vi "BT-Android_AE_sub.vi"(5 "mode":T1, 6 "timeout (10sec)":u32=10000, 7 "End Write on Termination Character?":bool, 8 "error in (no error)":errorcluster, 10 "send data":string, 11 "VISA resource name":refnum<visa-resource-name>="COM13") -> (0 "error IO":errorcluster, 2 "timeout?":bool=TRUE)   [LabVIEW 2016, in "BT-Android_interface.lvlib"]
uses:
  BT-Android_interface.lvlib
  mode.ctl
  <vilib>/Instr/_visa.llb/VISA Configure Serial Port (Instr).vi
panel:
  out "Bytes Remain":u32
  in  "Termination Character":u8=10 format="%.0x"
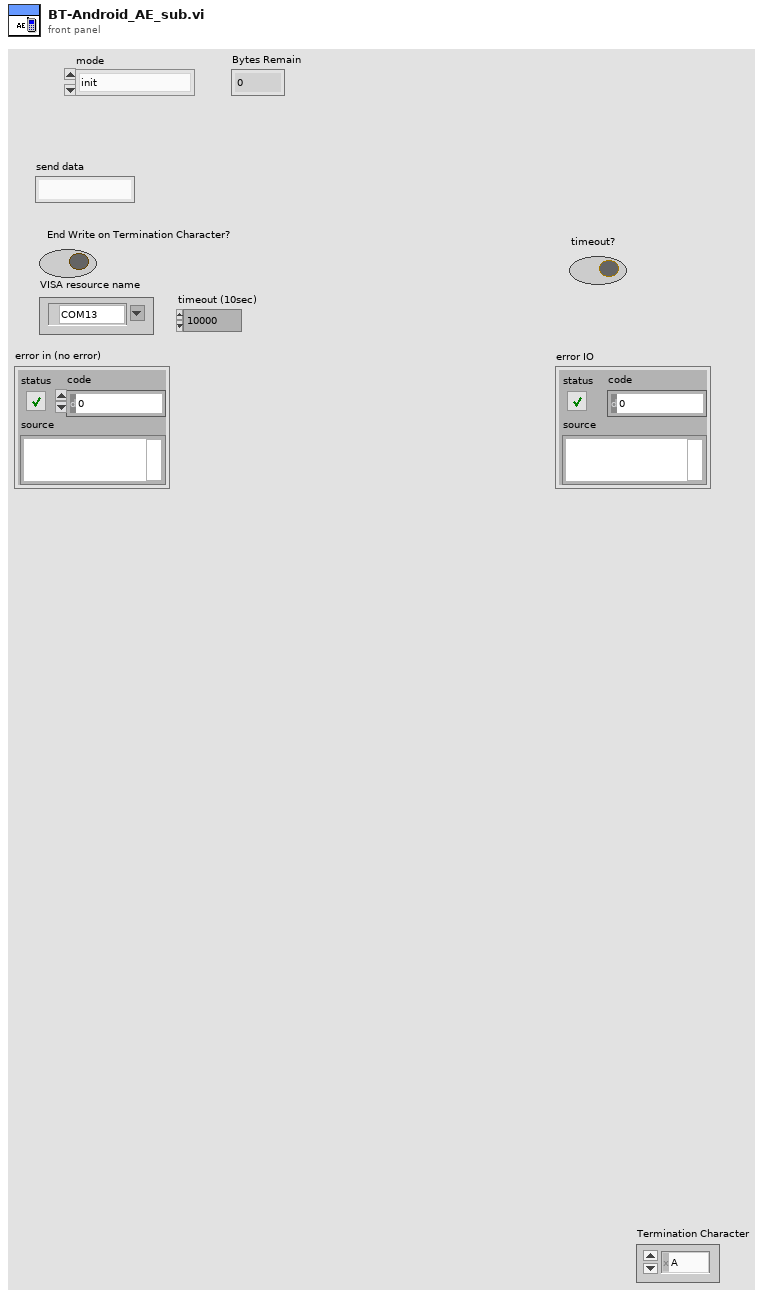
[diagram p1: front panel]
types:
  T1 = typedef "BT-Android_interface.lvlib/mode.ctl" = enum16{"init", "broadcast_data", "receive_data", "close"}
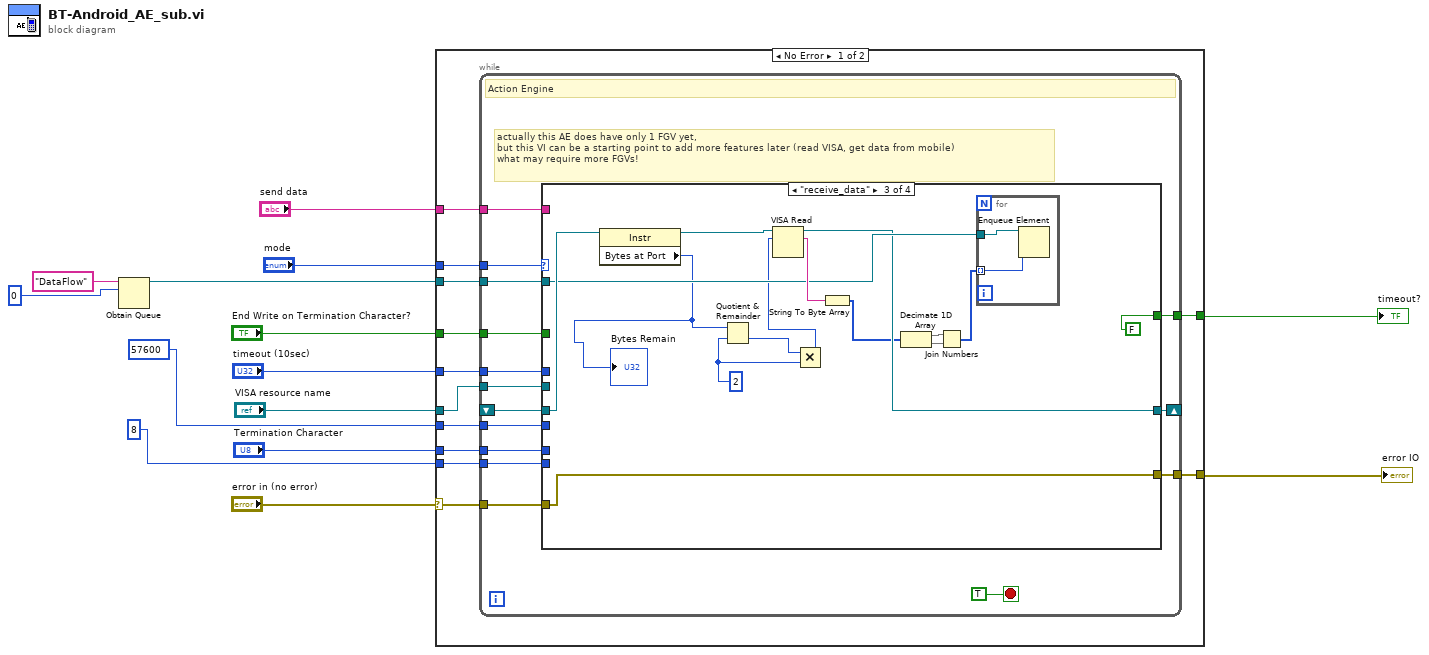
[diagram p0: block diagram]
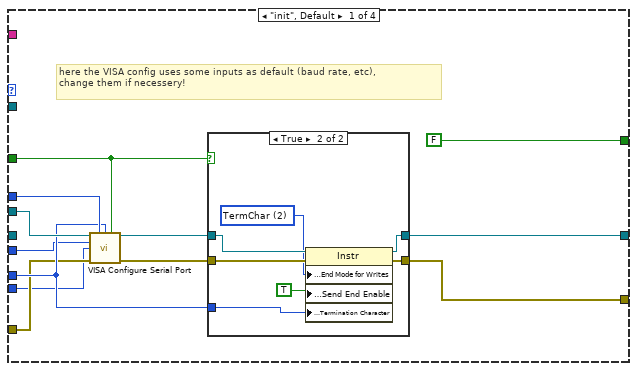
[diagram p2: hidden frame]
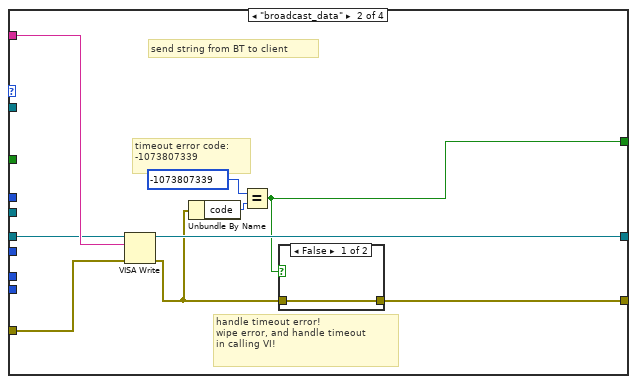
[diagram p4: hidden frame]
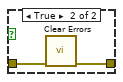
[diagram p5: hidden frame]
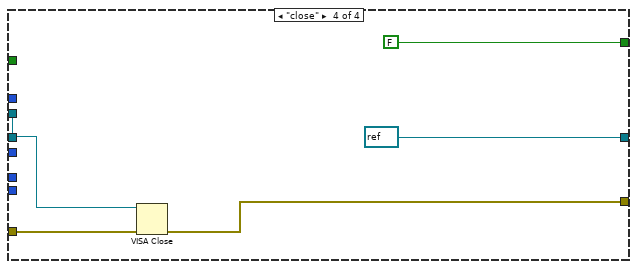
[diagram p6: hidden frame]
diagram:
  n1 = Obtain Queue(name (unnamed)="DataFlow", element data type=u16 0) -> (queue out=w3:refnum<queue>)  [unwired: 3 in, 2 out]
  n2 = case shown="No Error" "error in (no error)" {
    selector: "error in (no error)" -> [w26 w98]
    tunnel: [w22 w98] -> w13
    tunnel: "mode" -> [w25 _]
    tunnel: "End Write on Termination Character?" -> [w24 _]
    tunnel: "timeout (10sec)" -> [w23 _]
    tunnel: "VISA resource name" -> [w18 _]
    tunnel: "Termination Character" -> [w21 _]
    tunnel: "send data" -> [w20 _]
    tunnel: [w19 FALSE] -> w6
    tunnel: w3 -> [w17 _]
    tunnel: u32 57600 -> [w16 _]
    tunnel: 8 -> [w15 _]
    frame No Error {
      n3 = while {
        tunnel: w26 -> [w40]
        tunnel: w25 -> [w39]
        tunnel: w24 -> [w38]
        tunnel: w23 -> [w37]
        shift-right: [w36] -> _
        shift-left: _ -> [w30]
        tunnel: [w35] -> w22
        tunnel: w21 -> [w34]
        tunnel: w20 -> [w33]
        tunnel: [w32] -> w19
        tunnel: w18 -> [w31]
        tunnel: w17 -> [w29]
        tunnel: w16 -> [w28]
        tunnel: w15 -> [w27]
        stop <- TRUE stop-if-true
        # "actually this AE does have only 1 FGV yet, \nbut this VI can be a starting point to add more features later (read VISA, get data from mobile)\nwhat may require more FGVs!"
        # "Action Engine"
        n4 = case shown="\"receive_data\"" w39 {
          tunnel: w40 -> [w46 w71 w83 w96]
          tunnel: w38 -> [w44 _ _ _]
          tunnel: w37 -> [w51 _ _ _]
          tunnel: w31 -> [w50 _ _ w94]
          tunnel: [w49 w70 w84 refnum<visa-resource-name> refnum ("VISA resource name out")] -> w36
          tunnel: [w48 w68 w83 w95] -> w35
          tunnel: w34 -> [w47 _ _ _]
          tunnel: w33 -> [_ w69 _ _]
          tunnel: [FALSE w64 FALSE FALSE] -> w32
          tunnel: w30 -> [_ w63 w89 _]
          tunnel: w29 -> [_ _ w86 _]
          tunnel: w28 -> [w43 _ _ _]
          tunnel: w27 -> [w42 _ _ _]
          frame "init", Default {
            # "here the VISA config uses some inputs as default (baud rate, etc),\nchange them if necessery!"
            n5 = call-poly "VISA Configure Serial Port"("VISA resource name"=w50, "timeout (10sec)"=w51, "termination char\n(0xA = '\\n' = LF)"=w47, "Enable Termination\nChar (T)"=w44, "baud rate (9600)"=w43, "data bits (8)"=w42, "error in (no error)"=w46) -> ("VISA resource name out"=w52:refnum<visa-resource-name>, "error out"=w53:errorcluster)  [unwired: 3 in, 4 out]
            n6 = case shown="True" w44 {
              tunnel: w52 -> [w54 w62]
              tunnel: w53 -> [w55 w61]
              tunnel: [w54 w60] -> w49
              tunnel: [w55 w59] -> w48
              tunnel: w47 -> [_ w57]
              frame False {
              }
              frame True {
                w58 = u16 2 items=["None", "LastBit", "TermChar", "Break"] ("Serial Settings:Serial End Mode for Writes")
                n7 = property class="Instr"(reference=w62, error in=w61, "Serial Settings:End Mode for Writes"=w58, "Message Based Settings:Send End Enable"=TRUE, "Message Based Settings:Termination Character"=w57) -> (reference out=w60:refnum<visa-resource-name>, error out=w59:errorcluster)
              }
            }
          }
          frame "broadcast_data" {
            # "send string from BT to client"
            # "handle timeout error!\nwipe error, and handle timeout\nin calling VI!"
            # "timeout error code:\n-1073807339"
            n8 = VISA Write(VISA resource name=w63, write buffer=w69, error in (no error)=w71) -> (VISA resource name out=w70:refnum<visa-resource-name>, error out=w67:errorcluster)  [unwired: 1 out]
            n9 = Unbundle By Name(w67) -> ("code"=w66:i32)
            n10 = Equal?(x=-1073807339 ("code"), y=w66) -> (x = y?=w64:bool)
            n11 = case shown="False" w64 {
              tunnel: w67 -> [w72 w74]
              tunnel: [w72 w73] -> w68
              frame False {
              }
              frame True {
                n12 = call <vilib>:"Clear Errors.vi"("error in (no error)"=w74) -> ("error out"=w73:errorcluster)  [unwired: 5 in, 1 out]
              }
            }
          }
          frame "receive_data" {
            w77 = u32 2 ("y")
            n13 = property class="Instr"(reference=w89) -> (reference out=w88:refnum<visa-resource-name>, "Bytes at Port"=w75:u32)  [unwired: 1 in, 1 out]
            "Bytes Remain" <- w75
            n14 = Quotient & Remainder(x=w75, y=w77) -> (floor(x/y)=w78:u32)  [unwired: 1 out]
            n15 = Multiply(x=w78, y=w77) -> (x*y=w76:u32)
            n16 = VISA Read(VISA resource name=w88, byte count=w76) -> (VISA resource name out=w84:refnum<visa-resource-name>, read buffer=w87:string)  [unwired: 1 in, 2 out]
            n17 = String To Byte Array(string=w87) -> (unsigned byte array=w80:u8[])
            n18 = Decimate 1D Array(w80) -> (w82:u8[], w81:u8[])
            n19 = Join Numbers(hi=w82, lo=w81) -> ((hi.lo)=w79:u16[])
            n20 = for {
              tunnel: w79 -> [w91] mode=indexing
              tunnel: w86 -> [w90]
              n21 = Enqueue Element(queue=w90, element=w91) -> ()  [unwired: 2 in, 3 out]
            }
          }
          frame "close" {
            n22 = VISA Close(VISA resource name=w94, error in (no error)=w96) -> (error out=w95:errorcluster)
          }
        }
      }
    }
    frame Error {
    }
  }
  "error IO" <- w13
  "timeout?" <- w6
